vi "RT.vi"(1 "Ctl Refnum 2":refnum<vi>, 2 "Ctl Refnum":refnum<vi>, 5 "Cluster 3":T1, 6 "6517B":bool, 7 "簇":cluster{"开始温度":dbl, "结束温度":dbl, "变温速率":dbl}, 8 "error in (no error)":errorcluster caption="错误输入（无错误）", 9 "Cluster":T2={"电阻计地址"="USB0::0x0471::0x2826::QF71600867::INSTR", "电容计地址"="USB0::0x0471::0x2826::QF71600867::INSTR", "低温地址"="USB0::0x0471::0x2826::QF71600867::INSTR", "高温地址 2"="USB0::0x0471::0x2826::QF71600867::INSTR"}, 10 "文本":path, 11 "表格":path) -> (0 "错误输出":cluster{"状态":bool, "代码":i32, "源":string})   [LabVIEW 2017]
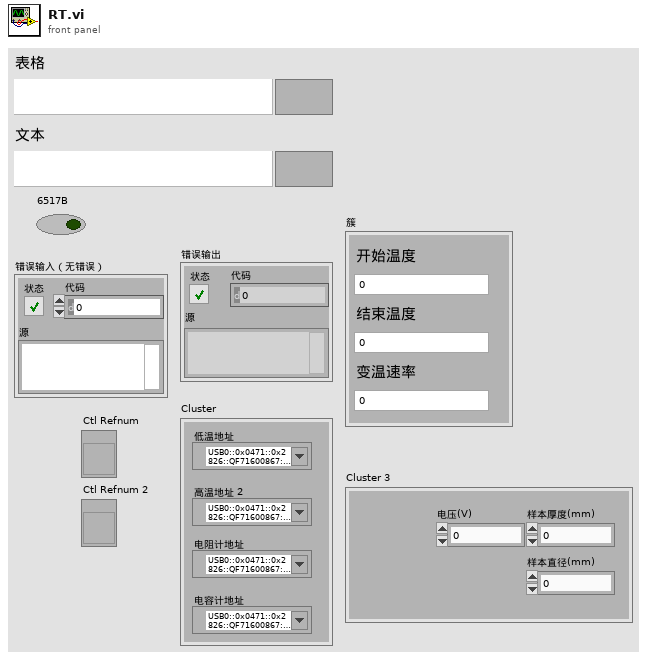
[diagram p1: front panel]
types:
  T1 = cluster{"电压(V)":dbl, "样本直径(mm)":dbl, "样本厚度(mm)":dbl}
  T2 = cluster{"电阻计地址":refnum<visa-resource-name>, "电容计地址":refnum<visa-resource-name>, "低温地址":refnum<visa-resource-name>, "高温地址 2":refnum<visa-resource-name>}
  T3 = enum16{"open", "replace", "create", "open or create", "replace or create", "replace or create with confirmation"}
  T4 = cluster{"电容计地址":refnum<visa-resource-name>, "低温地址":refnum<visa-resource-name>, "高温地址 2":refnum<visa-resource-name>}
  T5 = cluster{"Array":string[][], "error out":errorcluster}
  T6 = cluster{"簇":cluster{"开始温度":dbl, "结束温度":dbl, "变温速率":dbl}, "Cluster 3":cluster{"电压(V)":dbl, "样本直径(mm)":dbl, "样本厚度(mm)":dbl}}
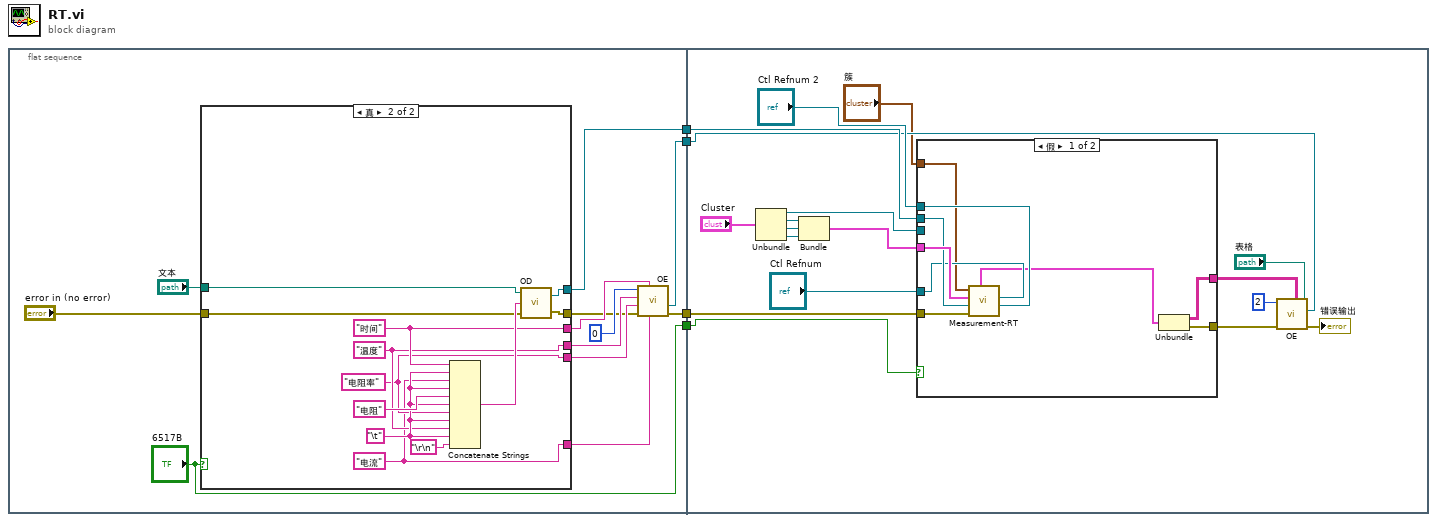
[diagram p0: block diagram]
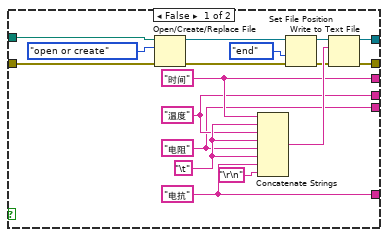
[diagram p2: hidden frame]
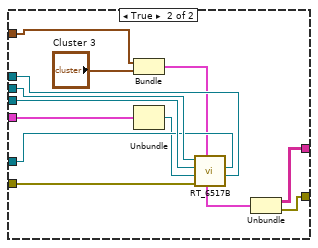
[diagram p3: hidden frame]
diagram:
  n1 = flat-sequence {
    tunnel: [w6] -> w4
    tunnel: [w13] -> w3
    tunnel: ["6517B"] -> w2
    tunnel: [w5] -> w1
    tunnel: w4 -> [w62]
    tunnel: w3 -> [w60]
    tunnel: w2 -> [w55]
    tunnel: w1 -> [w48]
    frame #0 {
      n2 = case shown="真" "6517B" {
        tunnel: "error in (no error)" -> [w25 w40]
        tunnel: "文本" -> [w23 w41]
        tunnel: [w22 w39] -> w7
        tunnel: [w21 w38] -> w13
        tunnel: [w20 w37] -> w11
        tunnel: [w19 w36] -> w10
        tunnel: [w18 w35] -> w9
        tunnel: [w17 w34] -> w8
        frame False {
          w17 = "电抗" ("字符串")
          w18 = "电阻" ("字符串")
          w19 = "温度" ("字符串")
          w28 = "\t"
          w20 = "时间" ("字符串")
          n3 = Open/Create/Replace File(file path (use dialog)=w23, error in=w25, operation (0:open)=T3."open or create" ("操作(0:open)")) -> (refnum out=w31:refnum<file>, error out=w32:errorcluster)  [unwired: 4 out]
          n4 = Concatenate Strings(w20, w28, w19, w28, w18, w28, w17, "\r\n") -> (w33:string)
          n5 = Set File Position(refnum=w31, from (0:start)=enum16{"start", "end", "current"}."end" ("自（0:起始）"), error in=w32) -> (refnum out=w30:refnum<file>, error out=w29:errorcluster)  [unwired: 1 out]
          n6 = Write to Text File(file (use dialog)=w30, text=w33, error in=w29) -> (refnum out=w21:refnum<file>, error out=w22:errorcluster)  [unwired: 2 out]
        }
        frame True {
          w36 = "温度" ("字符串")
          w35 = "电阻率" ("字符串")
          w34 = "电流"
          w44 = "\t"
          w37 = "时间" ("字符串")
          n7 = Concatenate Strings(w37, w44, w34, w44, "电阻", w44, w35, w44, w36, w44, "\r\n") -> (w42:string)
          n8 = call "OD.vi"("error in (no error)"=w40, "字符串"=w42, "路径"=w41) -> ("error out"=w39:errorcluster, "引用句柄输出"=w38:refnum<file>)
        }
      }
      n9 = call "OE.vi"("String 4"=w8, "String"=w11, "error in (no error)"=w7, "String 3"=w9, "String 2"=w10, "Numeric"=0) -> ("error out"=w6:errorcluster, "report out"=w5:refnum<class "NI_report.lvclass">)  [unwired: 3 in, 1 out]
    }
    frame #1 {
      n10 = Unbundle("Cluster") -> ("电阻计地址"=w59:refnum<visa-resource-name>, "电容计地址"=w57:refnum<visa-resource-name>, "低温地址"=w58:refnum<visa-resource-name>, "高温地址 2"=w56:refnum<visa-resource-name>)
      n11 = Bundle("电容计地址"=w57, "低温地址"=w58, "高温地址 2"=w56) -> (w61:T4)  [unwired: 1 in]
      n12 = case shown="假" w55 {
        tunnel: w62 -> [w70 w79]
        tunnel: w61 -> [w72 w84]
        tunnel: [w66 w76] -> w51
        tunnel: w60 -> [w71 w83]
        tunnel: w59 -> [_ w85]
        tunnel: "簇" -> [w64 w74]
        tunnel: "Ctl Refnum" -> [w69 w82]
        tunnel: "Ctl Refnum 2" -> [w68 w81]
        tunnel: [w65 w77] -> w49
        frame False {
          n13 = call "Measurement-RT.vi"("Ctl Refnum 2"=w68, "Ctl Refnum"=w69, "error in (no error)"=w70, "BSFR"=w71, "Cluster 2"=w72, "簇"=w64) -> ("Cluster"=w67:T5)  [unwired: 5 in]
          n14 = Unbundle(w67) -> ("Array"=w65:string[][], "error out"=w66:errorcluster)
        }
        frame True {
          n15 = Bundle("簇"=w74, "Cluster 3"="Cluster 3") -> (w73:T6)  [unwired: 1 in]
          n16 = Unbundle(w84) -> ("低温地址"=w80:refnum<visa-resource-name>)  [unwired: 2 out]
          n17 = call "RT_6517B.vi"("Ctl Refnum 2"=w81, "Ctl Refnum"=w82, "簇 2"=w73, "error in (no error)"=w79, "Temp. Adr."=w80, "6517 Adr."=w85, "引用句柄输出"=w83) -> ("Cluster 2"=w78:T5)  [unwired: 4 in]
          n18 = Unbundle(w78) -> ("Array"=w77:string[][], "error out"=w76:errorcluster)
        }
      }
      n19 = call "OE.vi"("report in"=w48, "表格数据路径："="表格", "Array"=w49, "error in (no error)"=w51, "Numeric"=2) -> ("error out"=→"错误输出":errorcluster)  [unwired: 4 in, 2 out]
    }
  }
